vi "Untitled 7.vi"   [LabVIEW 2015]
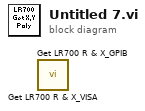
[diagram p0: block diagram]
diagram:
  n1 = call "Get LR700 R & X_VISA.vi"() -> ()  [unwired: 4 in, 4 out]
  n2 = call "Get LR700 R & X_GPIB.vi"() -> ()  [unwired: 5 in, 3 out]
